vi "Updater Perform Upgrade to Winows 7-2008.vi"(7 "Spartan Install Path":path, 8 "error in (no error)":errorcluster, 11 "Connection Refnum":T1) -> (0 "error out":errorcluster, 3 "Connection Refnum Out":T1)   [LabVIEW 2011]
uses:
  SI.LIB/ODBC/SQL Controls/Connection Refnum.ctl
  <vilib>/registry/registry.llb/Registry View.ctl
  <vilib>/registry/registry.llb/Read Registry Value Simple STR.vi
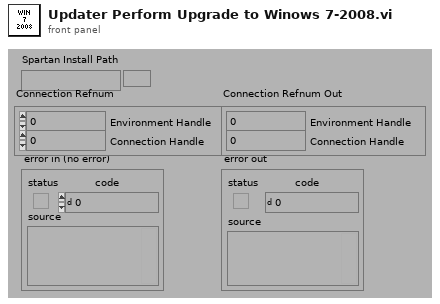
[diagram p1: front panel]
types:
  T1 = typedef "Connection Refnum.ctl" = cluster{"Environment Handle":i32, "Connection Handle":i32}
  T2 = typedef "Registry View.ctl" = u16
  T3 = typedef "Registry refnum.ctl" = refnum<k1>
  T4 = cluster{"numSubKeys":i32, "maxSubKeyLen":i32, "maxSubKeyClassLen":i32}
  T5 = typedef "Keyed Array.ctl" = cluster{"keys":string[], "values":string[]}
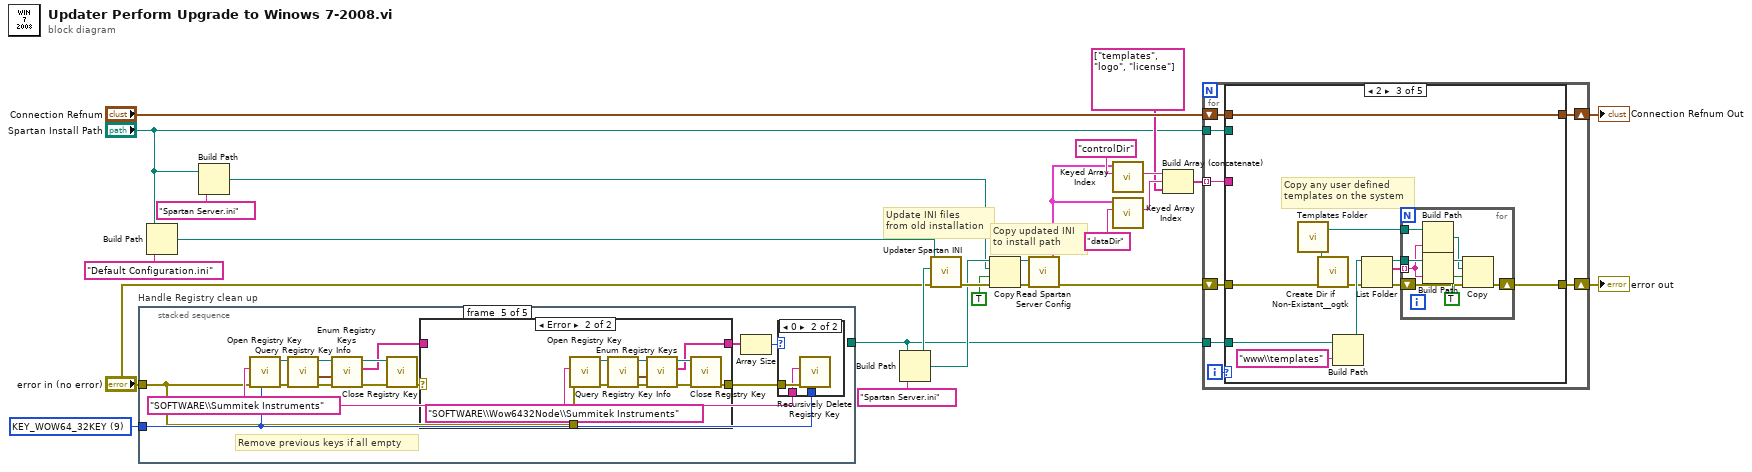
[diagram p0: block diagram]
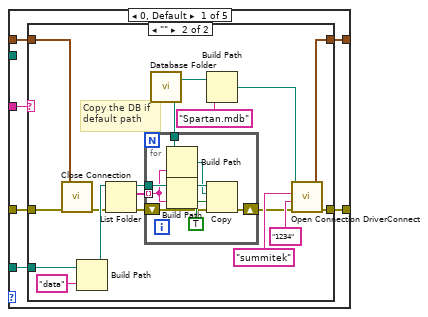
[diagram p2: hidden frame]
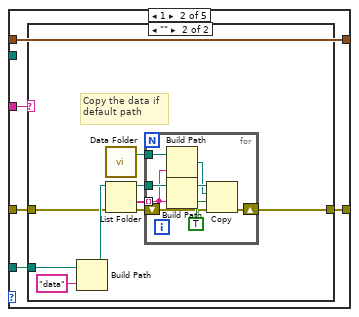
[diagram p4: hidden frame]
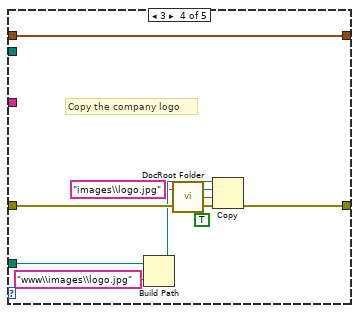
[diagram p6: hidden frame]
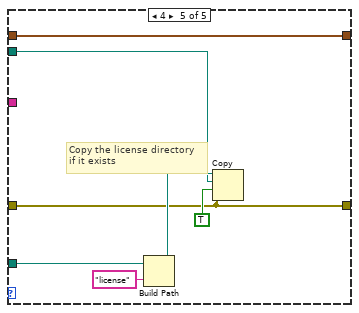
[diagram p7: hidden frame]
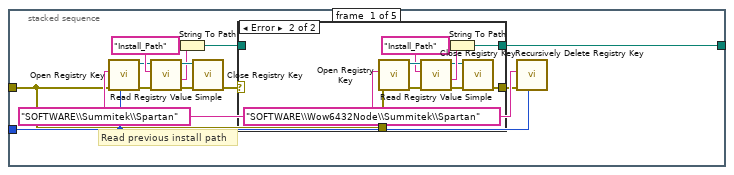
[diagram p8: hidden frame]
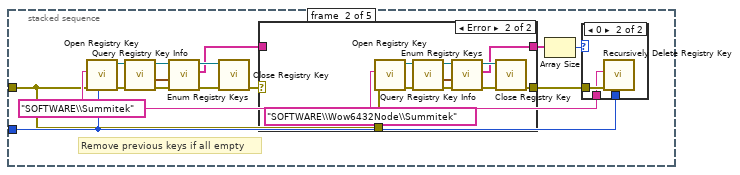
[diagram p10: hidden frame]
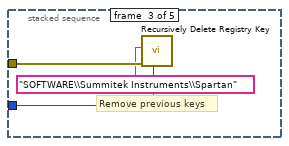
[diagram p13: hidden frame]
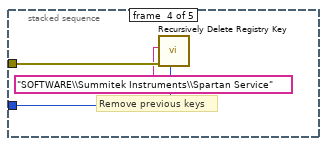
[diagram p14: hidden frame]
diagram:
  w3 = T2 9 items=["Default"=0, "KEY_WOW64_64KEY"=8, "KEY_WOW64_32KEY"=9] ("registry view")
  # "Copy updated INI\nto install path"
  # "Update INI files\nfrom old installation"
  n1 = stacked-sequence "Handle Registry clean up" {
    tunnel: "error in (no error)" -> [w28 w53 w84 w87 w88]
    tunnel: [w30 _ _ _ _] -> w11
    tunnel: w3 -> [w31 w56 w82 w85 w93]
    frame #0 {
      w38 = "SOFTWARE\\Summitek\\Spartan" ("subkey")
      # "Read previous install path"
      n2 = call <vilib>:"Open Registry Key.vi"("registry view"=w31, "error in (no error)"=w28, "subkey"=w38) -> ("error out"=w32:errorcluster, "refnum out"=w33:T3)  [unwired: 7 in]
      n3 = call-poly <vilib>:"Read Registry Value Simple.vi"("error in (no error)"=w32, "value"="Install_Path" ("subkey"), "refnum"=w33) -> ("error out"=w36:errorcluster, "String/Binary data"=w35:string, "refnum out"=w37:T3)  [unwired: 3 in, 1 out]
      n4 = String To Path(string=w35) -> (path=w29:path)
      n5 = call <vilib>:"Close Registry Key.vi"("error in (no error)"=w36, "refnum"=w37) -> ("error out"=w27:errorcluster)  [unwired: 5 in]
      n6 = case shown="Error" w27 {
        selector: w27 -> [w39 _]
        tunnel: [w40 w43] -> w30
        tunnel: w29 -> [w40 _]
        tunnel: w28 -> [_ w42]
        tunnel: [w39 w41] -> w26
        frame No Error {
        }
        frame Error {
          n7 = call <vilib>:"Open Registry Key.vi"("error in (no error)"=w42, "subkey"="SOFTWARE\\Wow6432Node\\Summitek\\Spartan") -> ("error out"=w50:errorcluster, "refnum out"=w49:T3)  [unwired: 8 in]
          n8 = call-poly <vilib>:"Read Registry Value Simple.vi"("error in (no error)"=w50, "value"="Install_Path" ("subkey"), "refnum"=w49) -> ("error out"=w46:errorcluster, "String/Binary data"=w47:string, "refnum out"=w45:T3)  [unwired: 3 in, 1 out]
          n9 = String To Path(string=w47) -> (path=w43:path)
          n10 = call <vilib>:"Close Registry Key.vi"("error in (no error)"=w46, "refnum"=w45) -> ("error out"=w41:errorcluster)  [unwired: 5 in]
        }
      }
      n11 = call "Recursively Delete Registry Key.vi"("Registry View"=w31, "error in (no error)"=w26, "Subkey"=w38) -> ()  [unwired: 8 in, 1 out]
    }
    frame #1 {
      w65 = "SOFTWARE\\Summitek" ("subkey")
      # "Remove previous keys if all empty"
      n12 = call <vilib>:"Open Registry Key.vi"("registry view"=w56, "error in (no error)"=w53, "subkey"=w65) -> ("error out"=w60:errorcluster, "refnum out"=w61:T3)  [unwired: 7 in]
      n13 = call <vilib>:"Query Registry Key Info.vi"("error in (no error)"=w60, "refnum"=w61) -> ("error out"=w58:errorcluster, "refnum out"=w59:T3, "subkey info"=w57:T4)  [unwired: 5 in, 2 out]
      n14 = call <vilib>:"Enum Registry Keys.vi"("error in (no error)"=w58, "subkey info"=w57, "refnum"=w59) -> ("error out"=w64:errorcluster, "subkeys"=w52:string[], "refnum out"=w63:T3)  [unwired: 6 in]
      n15 = call <vilib>:"Close Registry Key.vi"("error in (no error)"=w64, "refnum"=w63) -> ("error out"=w55:errorcluster)  [unwired: 5 in]
      n16 = case shown="Error" w55 {
        selector: w55 -> [w66 _]
        tunnel: [w67 w74] -> w51
        tunnel: w52 -> [w67 _]
        tunnel: [w66 w69] -> w54
        tunnel: w53 -> [_ w68]
        frame No Error {
        }
        frame Error {
          n17 = call <vilib>:"Open Registry Key.vi"("error in (no error)"=w68, "subkey"="SOFTWARE\\Wow6432Node\\Summitek") -> ("error out"=w72:errorcluster, "refnum out"=w71:T3)  [unwired: 8 in]
          n18 = call <vilib>:"Query Registry Key Info.vi"("error in (no error)"=w72, "refnum"=w71) -> ("error out"=w73:errorcluster, "refnum out"=w70:T3, "subkey info"=w77:T4)  [unwired: 5 in, 2 out]
          n19 = call <vilib>:"Enum Registry Keys.vi"("error in (no error)"=w73, "subkey info"=w77, "refnum"=w70) -> ("error out"=w76:errorcluster, "subkeys"=w74:string[], "refnum out"=w75:T3)  [unwired: 6 in]
          n20 = call <vilib>:"Close Registry Key.vi"("error in (no error)"=w76, "refnum"=w75) -> ("error out"=w69:errorcluster)  [unwired: 5 in]
        }
      }
      n21 = Array Size(array=w51) -> (size(s)=w62:i32)
      n22 = case shown="0" w62 {
        tunnel: w54 -> [_ w81]
        tunnel: w65 -> [_ w80]
        tunnel: w56 -> [_ w79]
        frame Default {
        }
        frame 0 {
          n23 = call "Recursively Delete Registry Key.vi"("Registry View"=w79, "error in (no error)"=w81, "Subkey"=w80) -> ()  [unwired: 8 in, 1 out]
        }
      }
    }
    frame #2 {
      # "Remove previous keys"
      n24 = call "Recursively Delete Registry Key.vi"("Registry View"=w82, "error in (no error)"=w84, "Subkey"="SOFTWARE\\Summitek Instruments\\Spartan" ("subkey")) -> ()  [unwired: 8 in, 1 out]
    }
    frame #3 {
      # "Remove previous keys"
      n25 = call "Recursively Delete Registry Key.vi"("Registry View"=w85, "error in (no error)"=w87, "Subkey"="SOFTWARE\\Summitek Instruments\\Spartan Service" ("subkey")) -> ()  [unwired: 8 in, 1 out]
    }
    frame #4 {
      w102 = "SOFTWARE\\Summitek Instruments" ("subkey")
      # "Remove previous keys if all empty"
      n26 = call <vilib>:"Open Registry Key.vi"("registry view"=w93, "error in (no error)"=w88, "subkey"=w102) -> ("error out"=w97:errorcluster, "refnum out"=w98:T3)  [unwired: 7 in]
      n27 = call <vilib>:"Query Registry Key Info.vi"("error in (no error)"=w97, "refnum"=w98) -> ("error out"=w95:errorcluster, "refnum out"=w96:T3, "subkey info"=w94:T4)  [unwired: 5 in, 2 out]
      n28 = call <vilib>:"Enum Registry Keys.vi"("error in (no error)"=w95, "subkey info"=w94, "refnum"=w96) -> ("error out"=w101:errorcluster, "subkeys"=w90:string[], "refnum out"=w100:T3)  [unwired: 6 in]
      n29 = call <vilib>:"Close Registry Key.vi"("error in (no error)"=w101, "refnum"=w100) -> ("error out"=w92:errorcluster)  [unwired: 5 in]
      n30 = case shown="Error" w92 {
        selector: w92 -> [w104 _]
        tunnel: [w103 w111] -> w89
        tunnel: [w104 w106] -> w91
        tunnel: w90 -> [w103 _]
        tunnel: w88 -> [_ w105]
        frame No Error {
        }
        frame Error {
          n31 = call <vilib>:"Open Registry Key.vi"("error in (no error)"=w105, "subkey"="SOFTWARE\\Wow6432Node\\Summitek Instruments") -> ("error out"=w109:errorcluster, "refnum out"=w108:T3)  [unwired: 8 in]
          n32 = call <vilib>:"Query Registry Key Info.vi"("error in (no error)"=w109, "refnum"=w108) -> ("error out"=w110:errorcluster, "refnum out"=w107:T3, "subkey info"=w114:T4)  [unwired: 5 in, 2 out]
          n33 = call <vilib>:"Enum Registry Keys.vi"("error in (no error)"=w110, "subkey info"=w114, "refnum"=w107) -> ("error out"=w113:errorcluster, "subkeys"=w111:string[], "refnum out"=w112:T3)  [unwired: 6 in]
          n34 = call <vilib>:"Close Registry Key.vi"("error in (no error)"=w113, "refnum"=w112) -> ("error out"=w106:errorcluster)  [unwired: 5 in]
        }
      }
      n35 = Array Size(array=w89) -> (size(s)=w99:i32)
      n36 = case shown="0" w99 {
        tunnel: w91 -> [_ w118]
        tunnel: w102 -> [_ w117]
        tunnel: w93 -> [_ w116]
        frame Default {
        }
        frame 0 {
          n37 = call "Recursively Delete Registry Key.vi"("Registry View"=w116, "error in (no error)"=w118, "Subkey"=w117) -> ()  [unwired: 8 in, 1 out]
        }
      }
    }
  }
  n38 = Build Path(base path="Spartan Install Path", name or relative path="Default Configuration.ini") -> (appended path=w24:path)
  n39 = Build Path(base path="Spartan Install Path", name or relative path="Spartan Server.ini") -> (appended path=w19:path)
  n40 = Build Path(base path=w11, name or relative path="Spartan Server.ini") -> (appended path=w21:path)
  n41 = call "Updater Spartan INI.vi"("error in (no error)"="error in (no error)", "Spartan Server.ini"=w21, "Copy Keys From INI"=w24) -> ("error out"=w22:errorcluster)  [unwired: 7 in, 1 out]
  n42 = Copy(8:w22, 9:TRUE ("overwrite (F)"), 10:w19, 11:w21) -> (0:w17:errorcluster, 3:w16:path)  [unwired: 1 in, 1 out]
  n43 = call "Read Spartan Server Config.vi"("error in (no error)"=w17, "Config File Path (empty - use default)"=w16) -> ("error out"=w12:errorcluster, "Config Keys"=w14:T5)  [unwired: 4 in]
  n44 = call "Keyed Array Index.vi"("key"="controlDir", "array in"=w14) -> ("value"=w10:string)  [unwired: 2 in, 3 out]
  n45 = call "Keyed Array Index.vi"("key"="dataDir", "array in"=w14) -> ("value"=w9:string)  [unwired: 2 in, 3 out]
  n46 = Build Array (concatenate)(w10, w9, string[] ["templates", "logo", "license"]) -> (w8:string[])
  n47 = for {
    tunnel: w8 -> [w125] mode=indexing
    tunnel: w11 -> [w124]
    shift-right: [w121] -> w6
    shift-left: "Connection Refnum" -> [w122]
    shift-right: [w120] -> w5
    shift-left: w12 -> [w126]
    tunnel: "Spartan Install Path" -> [w119]
    i -> [w123]
    n48 = case shown="2" w123 {
      tunnel: w126 -> [w132 w164 w185 w206 w212]
      tunnel: w125 -> [w131 w163 _ _ _]
      tunnel: w124 -> [w130 w162 w193 w210 w217]
      tunnel: w122 -> [w129 w161 w192 w209 w216]
      tunnel: [w128 w161 w192 w209 w216] -> w121
      tunnel: [w127 w160 w191 w208 w212] -> w120
      tunnel: w119 -> [_ _ _ _ w211]
      frame 0, Default {
        n49 = case shown="\"\"" w131 {
          tunnel: w132 -> [w133 w138]
          tunnel: w130 -> [_ w146]
          tunnel: w129 -> [w134 w149]
          tunnel: [w134 w148] -> w128
          tunnel: [w133 w137] -> w127
          frame Default {
          }
          frame "" {
            # "Copy the DB if\ndefault path"
            n50 = call "Close Connection.vi"("error in (no error)"=w138, "Connection Refnum"=w149) -> ("error out"=w135:errorcluster)  [unwired: 5 out]
            n51 = Build Path(base path=w146, name or relative path="data") -> (appended path=w144:path)
            n52 = List Folder(path=w144, error in=w135) -> (path out=w142:path, filenames=w143:string[], error out=w147:errorcluster)  [unwired: 2 in, 1 out]
            n53 = call "Database Folder.vi"() -> ("Data Folder"=w139:path)  [unwired: 3 in]
            n54 = for {
              shift-right: [w157] -> w136
              shift-left: w147 -> [w158]
              tunnel: w143 -> [w153] mode=indexing
              tunnel: w142 -> [w156]
              tunnel: w139 -> [w154]
              n55 = Build Path(base path=w154, name or relative path=w153) -> (appended path=w152:path)
              n56 = Build Path(base path=w156, name or relative path=w153) -> (appended path=w155:path)
              n57 = Copy(8:w158, 9:TRUE ("overwrite (F)"), 10:w152, 11:w155) -> (0:w157:errorcluster)  [unwired: 1 in, 2 out]
            }
            n58 = Build Path(base path=w139, name or relative path="Spartan.mdb" ("Username (\"\")")) -> (appended path=w140:path)
            n59 = call "Open Connection DriverConnect.vi"("error in (no error)"=w136, "Password (\"\")"="1234" ("Username (\"\")"), "Username (\"\")"="summitek" ("Username (\"\")"), "ODBC Database (\"\")"=w140) -> ("error out"=w137:errorcluster, "Connection Refnum"=w148:T1)  [unwired: 3 out]
          }
        }
      }
      frame 1 {
        n60 = case shown="\"\"" w163 {
          tunnel: w164 -> [w165 w169]
          tunnel: w162 -> [_ w173]
          tunnel: [w165 w167] -> w160
          frame Default {
          }
          frame "" {
            # "Copy the data if\ndefault path"
            n61 = Build Path(base path=w173, name or relative path="data") -> (appended path=w171:path)
            n62 = call "Data Folder.vi"() -> ("Data Folder"=w166:path)  [unwired: 3 in]
            n63 = List Folder(path=w171, error in=w169) -> (path out=w170:path, folder names=w168:string[], error out=w174:errorcluster)  [unwired: 2 in, 1 out]
            n64 = for {
              shift-right: [w180] -> w167
              shift-left: w174 -> [w181]
              tunnel: w168 -> [w177] mode=indexing
              tunnel: w170 -> [w179]
              tunnel: w166 -> [w175]
              n65 = Build Path(base path=w175, name or relative path=w177) -> (appended path=w176:path)
              n66 = Build Path(base path=w179, name or relative path=w177) -> (appended path=w178:path)
              n67 = Copy(8:w181, 9:TRUE ("overwrite (F)"), 10:w176, 11:w178) -> (0:w180:errorcluster)  [unwired: 1 in, 2 out]
            }
          }
        }
      }
      frame 2 {
        # "Copy any user defined\ntemplates on the system"
        n68 = call "Templates Folder.vi"() -> ("Templates Folder"=w183:path)  [unwired: 3 in]
        n69 = call "Create Dir if Non-Existant__ogtk.vi"("error in (no error)"=w185, "Directory Path"=w183) -> ("error out"=w184:errorcluster)  [unwired: 7 in, 2 out]
        n70 = Build Path(base path=w193, name or relative path="www\\templates") -> (appended path=w188:path)
        n71 = List Folder(path=w188, error in=w184) -> (path out=w187:path, filenames=w186:string[], error out=w190:errorcluster)  [unwired: 2 in, 1 out]
        n72 = for {
          shift-right: [w199] -> w191
          shift-left: w190 -> [w200]
          tunnel: w186 -> [w196] mode=indexing
          tunnel: w187 -> [w198]
          tunnel: w183 -> [w194]
          n73 = Build Path(base path=w194, name or relative path=w196) -> (appended path=w195:path)
          n74 = Build Path(base path=w198, name or relative path=w196) -> (appended path=w197:path)
          n75 = Copy(8:w200, 9:TRUE ("overwrite (F)"), 10:w195, 11:w197) -> (0:w199:errorcluster)  [unwired: 1 in, 2 out]
        }
      }
      frame 3 {
        # "Copy the company logo"
        n76 = Build Path(base path=w210, name or relative path="www\\images\\logo.jpg") -> (appended path=w205:path)
        n77 = call "DocRoot Folder.vi"("Relative Path (\"\" - Folder)"="images\\logo.jpg" ("name or relative path")) -> ("DocumentRoot Folder"=w204:path)  [unwired: 2 in]
        n78 = Copy(8:w206, 9:TRUE ("overwrite (F)"), 10:w204, 11:w205) -> (0:w208:errorcluster)  [unwired: 1 in, 2 out]
      }
      frame 4 {
        # "Copy the license directory\nif it exists"
        n79 = Build Path(base path=w217, name or relative path="license") -> (appended path=w214:path)
        n80 = Copy(8:w212, 9:TRUE ("overwrite (F)"), 10:w211, 11:w214) -> ()  [unwired: 1 in, 3 out]
      }
    }
  }
  "error out" <- w5
  "Connection Refnum Out" <- w6
